vi "PlayMusic.vi"(0 "reference in":refnum<class "MediaPlayer.lvclass">, 11 "Error In":errorcluster) -> (4 "reference out":refnum<class "MediaPlayer.lvclass">, 6 "Duration":dbl, 15 "Error Out":errorcluster)   [LabVIEW 2024, in "MediaPlayer.lvclass"]
uses:
  MediaPlayer.lvclass
  MediaPlayer.lvclass/MediaPlayer.ctl
  <vilib>/sound2/lvsound2.llb/Sound File Info (path).vi
panel:
  # "Connector Pane"
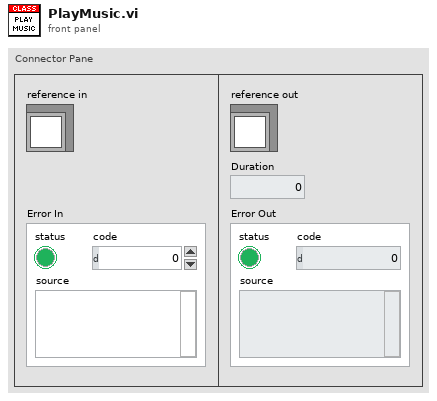
[diagram p1: front panel]
types:
  T1 = typedef "MediaPlayer.lvclass/ObjectAttributes.ctl" = cluster{"MediaPlayerData":T2}
  T2 = typedef "MediaPlayer.lvclass/MediaPlayer Data.ctl" = cluster{"Music List":path[], "Current Music Index":u16, "Song Handler":T3}
  T3 = typedef "Sound Output Task ID.ctl" = u32
  T4 = typedef "Sound Data Format.ctl" = cluster{"sample rate (S/s)":dbl, "number of channels":i32, "bits per sample":i32}
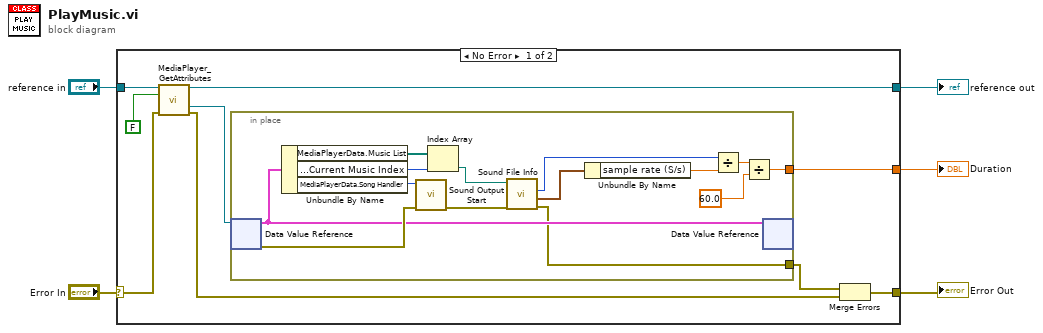
[diagram p0: block diagram]
diagram:
  n1 = case shown="No Error" "Error In" {
    selector: "Error In" -> [w13 w30]
    tunnel: [w8 w30] -> w4
    tunnel: [w12 w29] -> w2
    tunnel: "reference in" -> [w14 w29]
    tunnel: [w6 _] -> w1
    frame No Error {
      n2 = call "MediaPlayer_GetAttributes.vi"("reference in"=w14, "OnlyGetDvrReference(False)"=FALSE, "Error In"=w13) -> ("reference out"=w12:refnum<class "MediaPlayer.lvclass">, "DataRef"=w9:refnum<data-value>, "Error Out"=w10:errorcluster)  [unwired: 9 in, 1 out]
      n3 = in-place {
        in-place-border: [w22] -> w7
        in-place-border: [w15] -> w6
        n4 = in-place-dvr #1(w9) -> (w26:T1, w27:errorcluster)
        n5 = Unbundle By Name(w26) -> ("MediaPlayerData.Music List"=w24:path[], "MediaPlayerData.Current Music Index"=w25:u16, "MediaPlayerData.Song Handler"=w28:T3)
        n6 = call <vilib>:"Sound Output Start.vi"("error in (no error)"=w27, "task ID"=w28) -> ("error out"=w23:errorcluster)  [unwired: 8 in, 1 out]
        n7 = Index Array(array=w24, index=w25) -> (element=w21:path)
        n8 = call-poly <vilib>:"Sound File Info.vi"("error in (no error)"=w23, "path"=w21) -> ("error out"=w22:errorcluster, "sound format"=w20:T4, "total number of samples/ch"=w18:u32)  [unwired: 6 in, 1 out]
        n9 = Unbundle By Name(w20) -> ("sample rate (S/s)"=w19:dbl)
        n10 = Divide(x=w18, y=w19) -> (x/y=w17:dbl)
        n11 = Divide(x=w17, y=60.0) -> (x/y=w15:dbl)
        n12 = in-place-dvr #1(w26) -> ()  [unwired: 2 out]
      }
      n13 = Merge Errors(w7, w10) -> (w8:errorcluster)
    }
    frame Error {
    }
  }
  "Error Out" <- w4
  "reference out" <- w2
  "Duration" <- w1
